vi "Configure DMRS For Mapping Type B.vi"(4 "Max Length (1)":i32=1, 5 "Additional Position (0)":i32, 6 "Config Type (1)":i32=1, 7 "BWP (BWP0)":i32(ring) items=["BWP0"], 8 "error in (no error)":errorcluster, 9 "CC (1)":T1=1, 10 "Instance (1)":T2=1, 11 "VISA resource name":refnum<visa-resource-name>) -> (0 "error out":errorcluster, 3 "VISA resource name out":refnum<visa-resource-name>)   [LabVIEW 2020, in "Rohde&Schwarz CMWXP NR FR1 Measurement.lvlib"]
doc: "Configures the DM-RS for mapping type B. The settings apply to the <BWP> on carrier <no>.\n\nAttribute:\nRSCMWXPNRFR1M_ATTR_DMRS_FOR_MAPPING_TYPE_B\n\nRemote-control command:\nCONFigure:NRSub:MEAS<i>[:CC<no>]:BWPart:PUSCh:DMTB"
uses:
  <instrlib>/Rohde&Schwarz CMWXP NR FR1 Measurement/Rohde&Schwarz CMWXP NR FR1 Measurement.lvlib
  <instrlib>/Rohde&Schwarz CMWXP NR FR1 Measurement/Private/_Instance.ctl
  <instrlib>/Rohde&Schwarz CMWXP NR FR1 Measurement/Private/_Carrier Component.ctl
  <instrlib>/Rohde&Schwarz CMWXP NR FR1 Measurement/Private/rsidr_core.llb/rsidr_core.lvlib
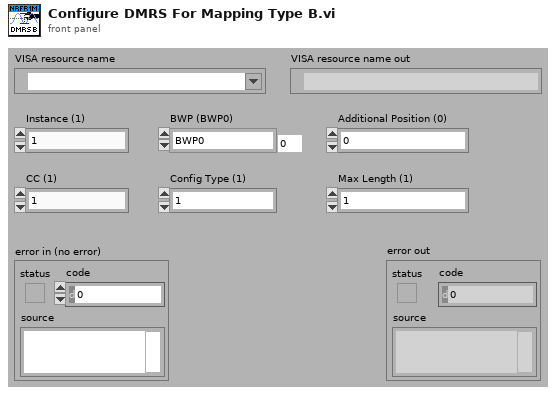
[diagram p1: front panel]
types:
  T1 = typedef "Rohde&Schwarz CMWXP NR FR1 Measurement.lvlib/_Carrier Component.ctl" = i32
  T2 = typedef "Rohde&Schwarz CMWXP NR FR1 Measurement.lvlib/_Instance.ctl" = i32
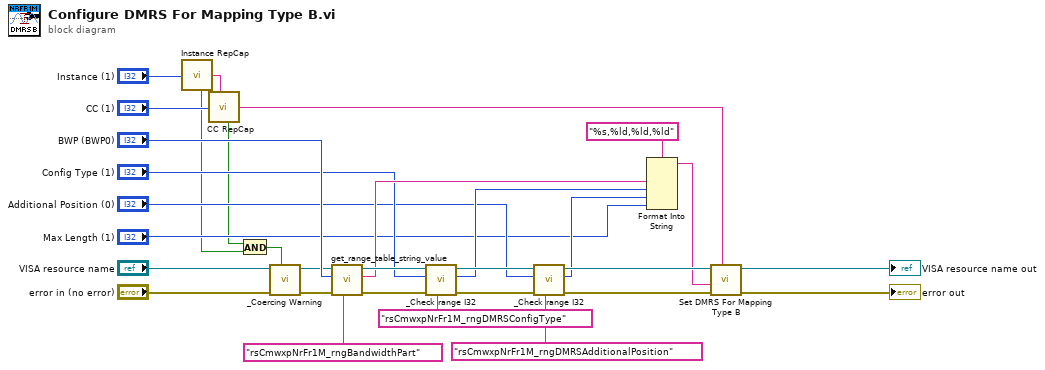
[diagram p0: block diagram]
diagram:
  n1 = call <instrlib>:"Instance RepCap.vi"("Instance In"="Instance (1)") -> ("In Range?"=w2:bool, "RepCap Identifier Out"=w31:string)  [unwired: 1 in]
  n2 = call <instrlib>:"CC RepCap.vi"("CC In"="CC (1)", "RepCap String In (\"\")"=w31) -> ("In Range?"=w1:bool, "RepCap Identifier Out"=w21:string)
  n3 = And(x=w1, y=w2) -> (x .and. y?=w3:bool)
  n4 = call <instrlib>:"_Coercing Warning.vi"("In Range?"=w3, "error in (no error)"="error in (no error)", "VISA resource name"="VISA resource name") -> ("error out"=w5:errorcluster, "VISA resource name out"=w4:refnum<visa-resource-name>)  [unwired: 7 in]
  n5 = call <instrlib>:"get_range_table_string_value.vi"("Range Table ID in"="rsCmwxpNrFr1M_rngBandwidthPart", "error in"=w5, "I32 input"="BWP (BWP0)", "VISA resource name"=w4) -> ("error out"=w30:errorcluster, "String Value out"=w19:string, "VISA resource name out"=w29:refnum<visa-resource-name>)  [unwired: 5 in]
  n6 = call <instrlib>:"_Check range I32.vi"("Range Table Identifier"="rsCmwxpNrFr1M_rngDMRSConfigType", "error in (no error)"=w30, "I32 Value In"="Config Type (1)", "VISA resource name"=w29) -> ("error out"=w26:errorcluster, "I32 Value Out"=w18:i32, "VISA resource name out"=w25:refnum<visa-resource-name>)  [unwired: 5 in]
  n7 = call <instrlib>:"_Check range I32.vi"("Range Table Identifier"="rsCmwxpNrFr1M_rngDMRSAdditionalPosition", "error in (no error)"=w26, "I32 Value In"="Additional Position (0)", "VISA resource name"=w25) -> ("error out"=w24:errorcluster, "I32 Value Out"=w17:i32, "VISA resource name out"=w23:refnum<visa-resource-name>)  [unwired: 5 in]
  n8 = Format Into String(format string="%s,%ld,%ld,%ld", w19, w18, w17, "Max Length (1)") -> (resulting string=w16:string)  [unwired: 2 in, 1 out]
  n9 = call "Set DMRS For Mapping Type B"("Repeated Capabilities"=w21, "error in (no error)"=w24, "DMRS For Mapping Type B ()"=w16, "instrument handle"=w23) -> ("error out"=→"error out":errorcluster, "instrument handle out"=→"VISA resource name out":refnum<visa-resource-name>)  [unwired: 6 in]
